vi "GV start acquisition.vi"() -> ()   [LabVIEW 2017]
panel:
  out "Start_acquisition":bool
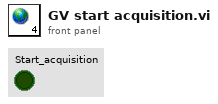
[diagram p1: front panel]
diagram:
